vi "Initialize Incoming Protection Signals.vi"(8 "error in (no error)":errorcluster, 9 "Incoming Signal Info In":T7 {"Signal Settings Out"."Protection Configuration"."CRC Channels"."Data Type" items=["Signed", "Unsigned", "IEEE Float"]}) -> (0 "error out":errorcluster, 1 "RT Incoming Signal Info":T1 {"Signal Settings Out"."Protection Configuration"."CRC Channels"."Data Type" items=["Signed", "Unsigned", "IEEE Float"]})   [LabVIEW 2019]
uses:
  Shared/Types/Incoming Signal Info.ctl
  Shared/Types/Exported Signal Settings.ctl
  Shared/Types/Exported Counter Settings.ctl
  Shared/Types/Exported Protection Settings.ctl
  Shared/Types/Protection Type.ctl
  Shared/Types/XNET Signal Configuration.ctl
  Shared/Types/RT_Incoming_Signal_Info.ctl
  Shared/Types/RT Exported Signal Settings.ctl
  Types/RT Protection Configuration.ctl
  <vilib>/xnet/xnet.llb/XNET Create Session (Conversion).vi
  Shared/Protection and Counter Support Shared.lvlib
  Protection and Counter Support Engine.lvlib
  <vilib>/NI VeriStand/Custom Device Tools/Custom Device Utility Library/Custom Device Utility Library.lvlib
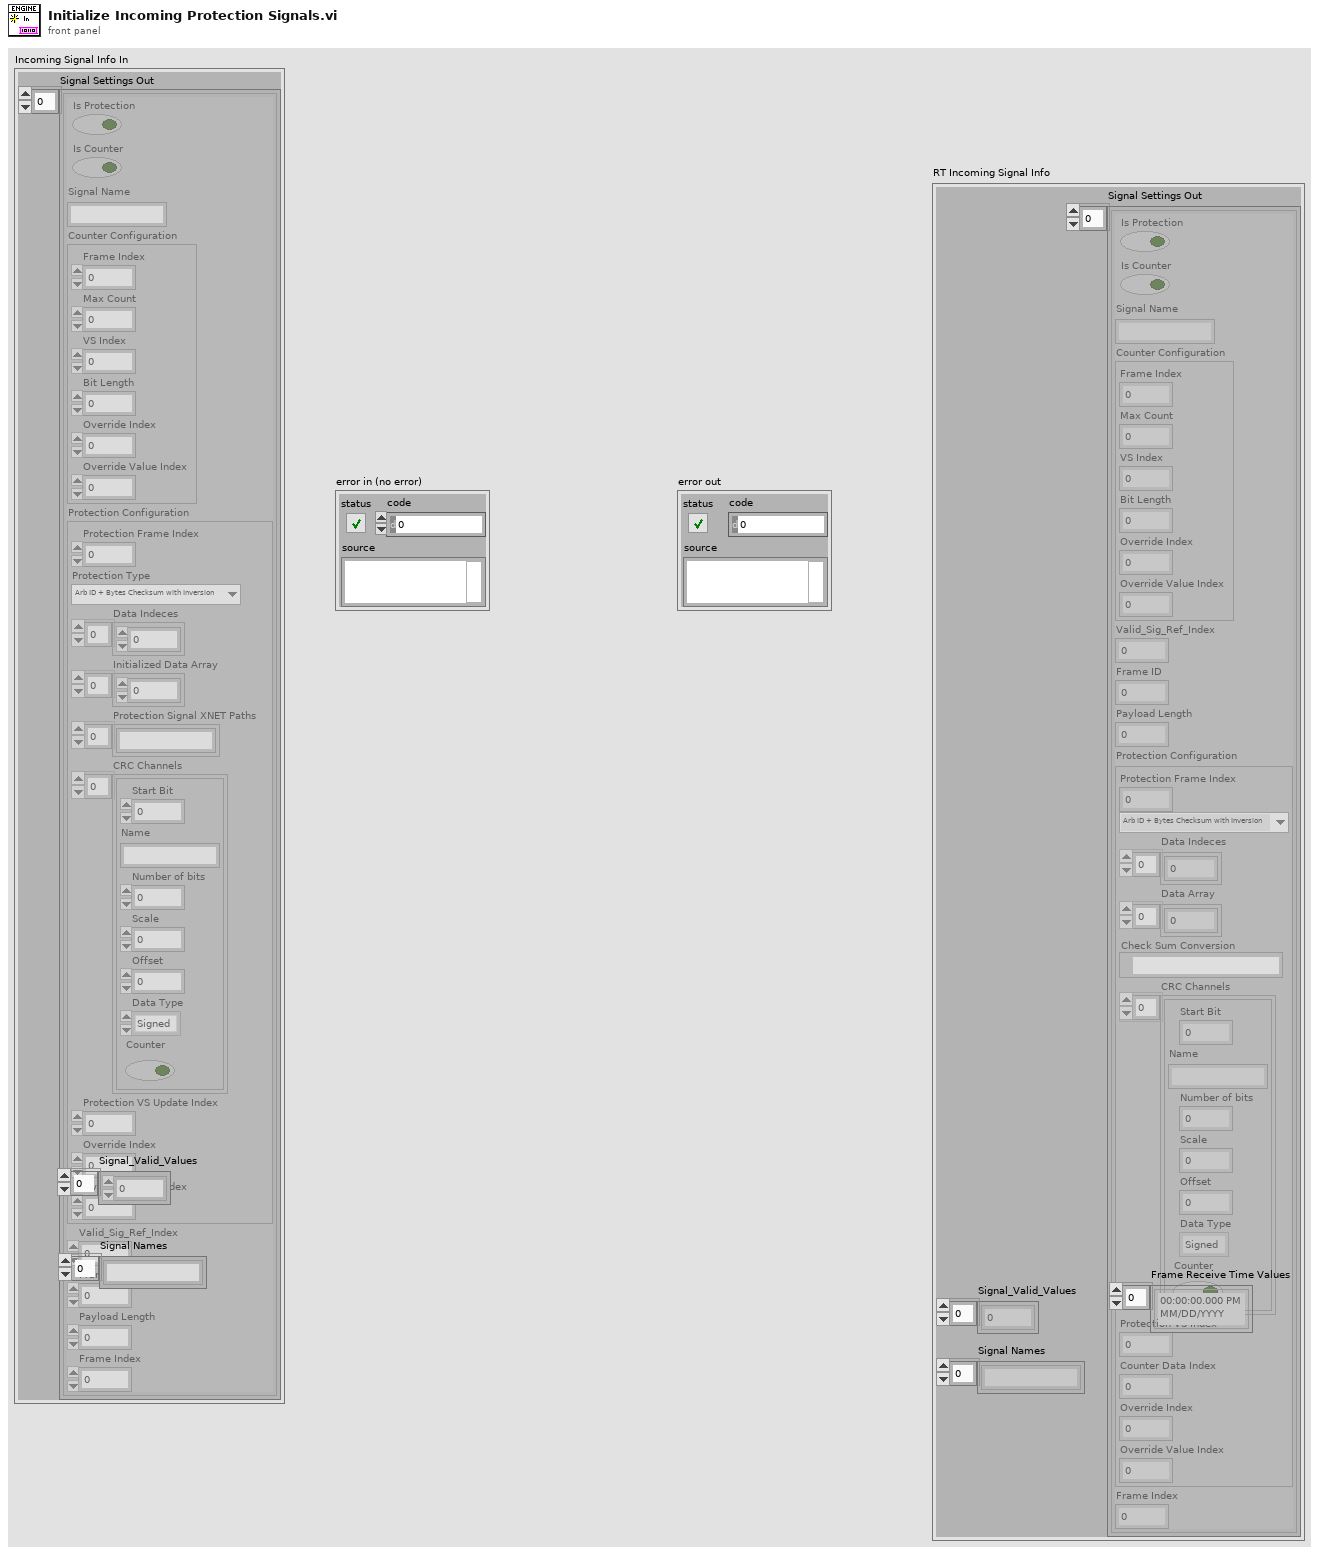
[diagram p1: front panel]
types:
  T1 = typedef "RT_Incoming_Signal_Info.ctl" = cluster{"Signal_Valid_Values":dbl[], "Signal Names":string[], "Signal Settings Out":T2[], "Frame Receive Time Values":timestamp[]}
  T2 = typedef "RT Exported Signal Settings.ctl" = cluster{"Is Protection":bool, "Is Counter":bool, "Signal Name":string, "Counter Configuration":T3, "Valid_Sig_Ref_Index":i32, "Frame ID":u32, "Payload Length":u32, "Protection Configuration":T4, "Frame Index":i32}
  T3 = typedef "Protection and Counter Support Shared.lvlib/Exported Counter Settings.ctl" = cluster{"Frame Index":i32, "Max Count":dbl, "VS Index":i32, "Bit Length":i64, "Override Index":i32, "Override Value Index":i32}
  T4 = typedef "Protection and Counter Support Engine.lvlib/RT Protection Configuration.ctl" = cluster{"Protection Frame Index":i32, "Protection Type":T5, "Data Indeces":i32[], "Data Array":dbl[], "Check Sum Conversion":refnum<k21>, "CRC Channels":T6[], "Protection VS Index":i32, "Counter Data Index":i32, "Override Index":i32, "Override Value Index":i32}
  T5 = typedef "Protection and Counter Support Shared.lvlib/Protection Type.ctl" = enum16{"Arb ID + Bytes Checksum with Inversion", "Arb ID + Bytes CRC with Inversion", "Reversed Raw Signal Checksum with Inversion", "Concatenated Two's Compliment"}
  T6 = typedef "Protection and Counter Support Shared.lvlib/XNET Signal Configuration.ctl" = cluster{"Start Bit":i32, "Name":string, "Number of bits":i32, "Scale":dbl, "Offset":dbl, "Data Type":u32, "Counter":bool}
  T7 = typedef "Incoming Signal Info.ctl" = cluster{"Signal Settings Out":T8[], "Signal_Valid_Values":dbl[], "Signal Names":string[]}
  T8 = typedef "Exported Signal Settings.ctl" = cluster{"Is Protection":bool, "Is Counter":bool, "Signal Name":string, "Counter Configuration":T3, "Protection Configuration":T9, "Valid_Sig_Ref_Index":i32, "Frame ID":u32, "Payload Length":u32, "Frame Index":i32}
  T9 = typedef "Protection and Counter Support Shared.lvlib/Exported Protection Settings.ctl" = cluster{"Protection Frame Index":i32, "Protection Type":T5, "Data Indeces":i32[], "Initialized Data Array":dbl[], "Protection Signal XNET Paths":string[], "CRC Channels":T6[], "Protection VS Update Index":i32, "Override Index":i32, "Override Value Index":i32}
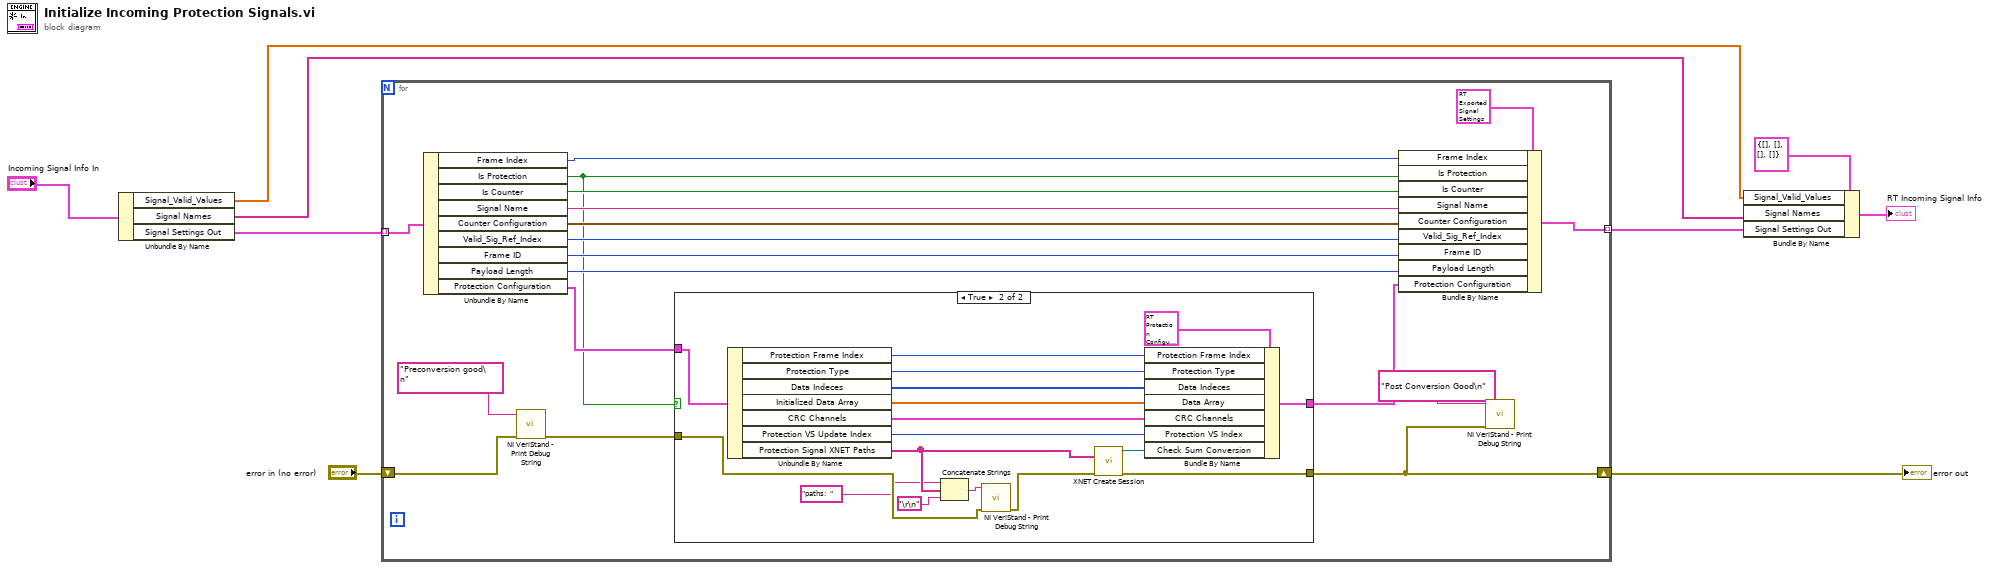
[diagram p0: block diagram]
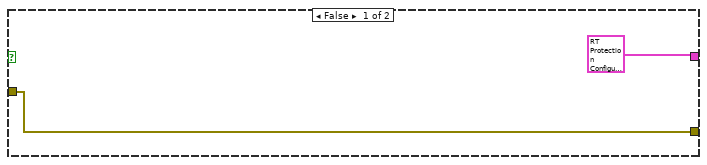
[diagram p2: hidden frame]
diagram:
  n1 = Unbundle By Name("Incoming Signal Info In") -> ("Signal_Valid_Values"=w2:dbl[], "Signal Names"=w1:string[], "Signal Settings Out"=w7:T8[])
  n2 = for {
    shift-right: [w16] -> w8
    shift-left: "error in (no error)" -> [w13]
    tunnel: w7 -> [w27] mode=indexing
    tunnel: [w17] -> w5 mode=indexing
    n3 = Unbundle By Name(w27) -> ("Frame Index"=w10:i32, "Is Protection"=w11:bool, "Is Counter"=w18:bool, "Signal Name"=w19:string, "Counter Configuration"=w20:T3, "Valid_Sig_Ref_Index"=w21:i32, "Frame ID"=w22:u32, "Payload Length"=w23:u32, "Protection Configuration"=w26:T9)
    n4 = call <vilib>:"NI VeriStand - Print Debug String.vi"("error in (no error)"=w13, "Message"="Preconversion good\n") -> ("error out"=w12:errorcluster)  [unwired: 9 in]
    n5 = case shown="True" w11 {
      tunnel: w26 -> [_ w46]
      tunnel: [T4 {"Protection Frame Index"=0, "Protection Type"=enum."Arb ID + Bytes Checksum with Inversion", "Data Indeces"=[], "Data Array"=[], "Check Sum Conversion"="", "CRC Channels"=[], "Protection VS Index"=0, "Counter Data Index"=0, "Override Index"=0, "Override Value Index"=0} ("Cluster") w37] -> w24
      tunnel: [w29 w36] -> w16
      tunnel: w12 -> [w29 w32]
      frame False {
      }
      frame True {
        n6 = Unbundle By Name(w46) -> ("Protection Frame Index"=w44:i32, "Protection Type"=w43:T5, "Data Indeces"=w42:i32[], "Initialized Data Array"=w41:dbl[], "CRC Channels"=w40:T6[], "Protection VS Update Index"=w39:i32, "Protection Signal XNET Paths"=w33:string[])
        n7 = Concatenate Strings("paths:  ", w33, "\r\n") -> (w35:string)
        n8 = call <vilib>:"NI VeriStand - Print Debug String.vi"("error in (no error)"=w32, "Message"=w35) -> ("error out"=w31:errorcluster)  [unwired: 9 in]
        n9 = call-poly <vilib>:"XNET Create Session.vi"("signal list"=w33, "error in (no error)"=w31) -> ("session out"=w38:refnum<k21>, "error out"=w36:errorcluster)  [unwired: 12 out]
        n10 = Bundle By Name(cluster=T4 {"Protection Frame Index"=0, "Protection Type"=enum."Arb ID + Bytes Checksum with Inversion", "Data Indeces"=[], "Data Array"=[], "Check Sum Conversion"="", "CRC Channels"=[], "Protection VS Index"=0, "Counter Data Index"=0, "Override Index"=0, "Override Value Index"=0} ("Cluster"), "Protection Frame Index"=w44, "Protection Type"=w43, "Data Indeces"=w42, "Data Array"=w41, "CRC Channels"=w40, "Protection VS Index"=w39, "Check Sum Conversion"=w38) -> (w37:T4)
      }
    }
    n11 = Bundle By Name(cluster=T2 {"Is Protection"=FALSE, "Is Counter"=FALSE, "Signal Name"="", "Counter Configuration"={"Frame Index"=0, "Max Count"=0.0, "VS Index"=0, "Bit Length"=0, "Override Index"=0, "Override Value Index"=0}, "Valid_Sig_Ref_Index"=0, "Frame ID"=0, "Payload Length"=0, "Protection Configuration"={"Protection Frame Index"=0, "Protection Type"=enum."Arb ID + Bytes Checksum with Inversion", "Data Indeces"=[], "Data Array"=[], "Check Sum Conversion"="", "CRC Channels"=[], "Protection VS Index"=0, "Counter Data Index"=0, "Override Index"=0, "Override Value Index"=0}, "Frame Index"=0} ("Signal Settings"), "Frame Index"=w10, "Is Protection"=w11, "Is Counter"=w18, "Signal Name"=w19, "Counter Configuration"=w20, "Valid_Sig_Ref_Index"=w21, "Frame ID"=w22, "Payload Length"=w23, "Protection Configuration"=w24) -> (w17:T2)
    n12 = call <vilib>:"NI VeriStand - Print Debug String.vi"("error in (no error)"=w16, "Message"="Post Conversion Good\n") -> ()  [unwired: 9 in, 1 out]
  }
  "error out" <- w8
  n13 = Bundle By Name(cluster=T1 {"Signal_Valid_Values"=[], "Signal Names"=[], "Signal Settings Out"=[], "Frame Receive Time Values"=[]} ("Incoming Signal Info Out 2"), "Signal_Valid_Values"=w2, "Signal Names"=w1, "Signal Settings Out"=w5) -> (→"RT Incoming Signal Info":T1)
